vi "Configure Math.vi"(0 "VISA resource name":refnum<visa-resource-name>, 1 "Operation (0:None)":i32(ring) items=["None", "Min/Max", "Relative", "dB", "dBm", "Compare", "MX+B"], 2 "Relative Offset (0)":dbl, 3 "dBm Resistance (600 Ohms)":i32(ring)=600 items=["2"=2, "4"=4, "8"=8, "16"=16, "50"=50, "75"=75, "93"=93, "110"=110, "124"=124, "125"=125, "135"=135, "150"=150, "250"=250, "300"=300, "500"=500, "600"=600, "800"=800, "900"=900, "1000"=1000, "1200"=1200, "8000"=8000], 5 "dB Reference Point (0V)":dbl, 7 "Upper Limit (1)":dbl=1.0, 9 "Lower Limit (-1)":dbl=-1.0, 11 "error in (no error)":errorcluster, 12 "Scale Factor M (1)":dbl=1.0, 13 "Offset Factor B (0)":dbl) -> (4 "VISA resource name out":refnum<visa-resource-name>, 15 "error out":errorcluster)   [LabVIEW 2021, in "GWInstek  GDM8351.lvlib"]
doc: "Configures the math functions available on the instrument."
uses:
  <instrlib>/GWInstek  GDM8351/GWInstek  GDM8351.lvlib
panel:
  # "Relative Function"
  # "MX+B"
  # "DB Measurements"
  # "Compare(Limit)"
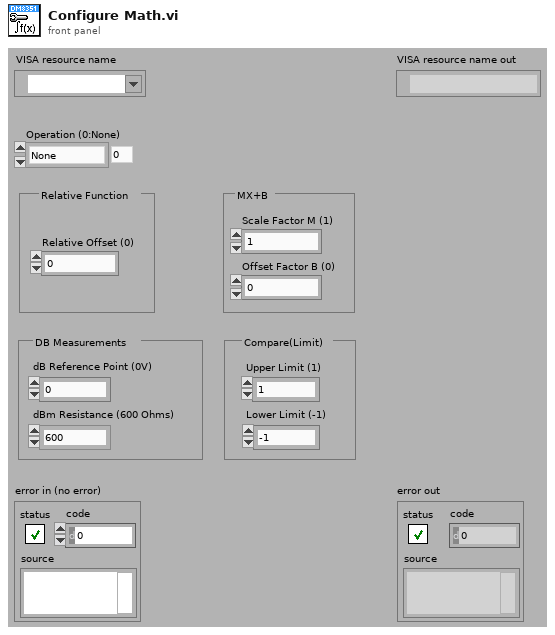
[diagram p1: front panel]
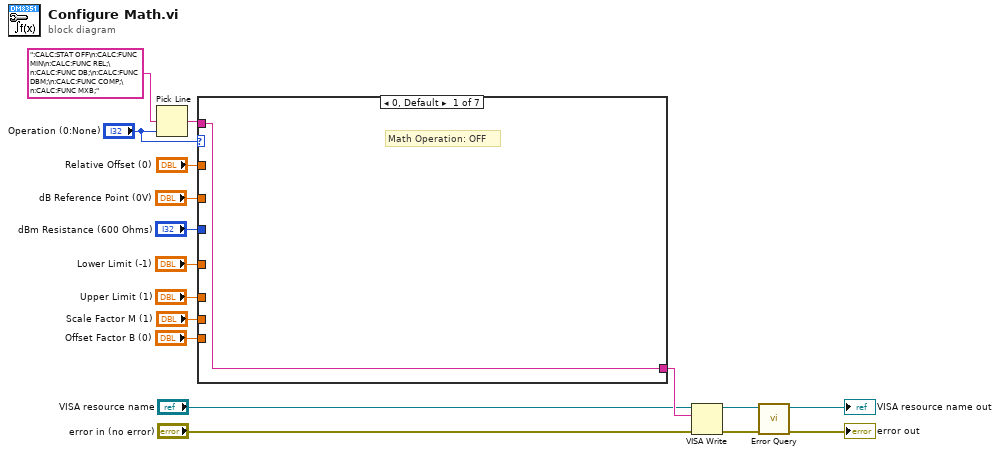
[diagram p0: block diagram]
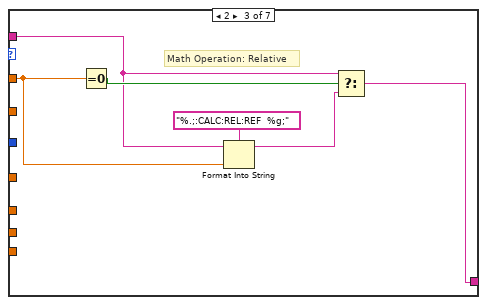
[diagram p3: hidden frame]
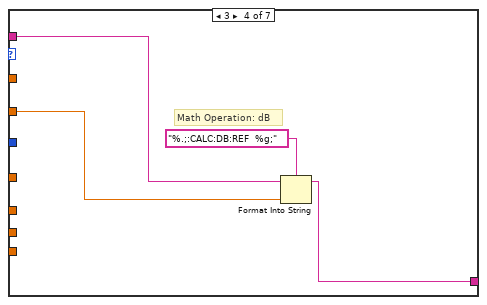
[diagram p4: hidden frame]
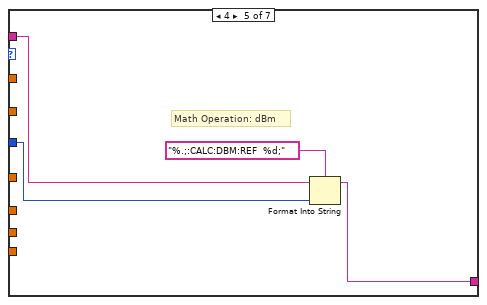
[diagram p5: hidden frame]
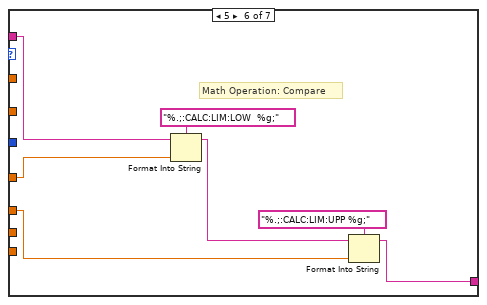
[diagram p6: hidden frame]
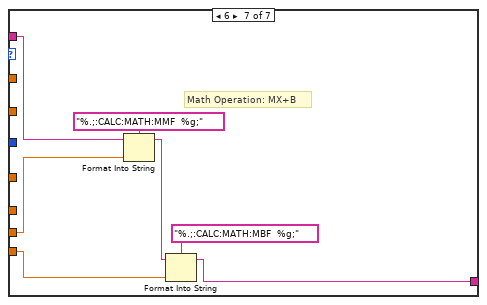
[diagram p7: hidden frame]
diagram:
  n1 = Pick Line(multi-line string=":CALC:STAT OFF\n:CALC:FUNC MIN\n:CALC:FUNC REL;\n:CALC:FUNC DB;\n:CALC:FUNC DBM;\n:CALC:FUNC COMP;\n:CALC:FUNC MXB;", line index="Operation (0:None)") -> (output string=w8:string)  [unwired: 1 in]
  n2 = case shown="0, Default" "Operation (0:None)" {
    tunnel: "Relative Offset (0)" -> [_ _ w22 _ _ _ _]
    tunnel: "dB Reference Point (0V)" -> [_ _ _ w29 _ _ _]
    tunnel: "dBm Resistance (600 Ohms)" -> [_ _ _ _ w31 _ _]
    tunnel: "Lower Limit (-1)" -> [_ _ _ _ _ w40 _]
    tunnel: "Upper Limit (1)" -> [_ _ _ _ _ w37 _]
    tunnel: "Scale Factor M (1)" -> [_ _ _ _ _ _ w47]
    tunnel: "Offset Factor B (0)" -> [_ _ _ _ _ _ w46]
    tunnel: w8 -> [w18 w19 w23 w28 w32 w39 w43]
    tunnel: [w18 w19 w20 w26 w30 w34 w41] -> w7
    frame 0, Default {
      # "Math Operation: OFF"
    }
    frame 1 {
      # "Math Operation: Min/Max"
    }
    frame 2 {
      # "Math Operation: Relative"
      n3 = Equal To 0?(x=w22) -> (x = 0?=w25:bool)
      n4 = Format Into String(format string="%.;:CALC:REL:REF  %g;", initial string=w23, w22) -> (resulting string=w21:string)  [unwired: 1 in, 1 out]
      n5 = Select(t=w23, s=w25, f=w21) -> (s? t:f=w20:string)
    }
    frame 3 {
      # "Math Operation: dB"
      n6 = Format Into String(format string="%.;:CALC:DB:REF  %g;", initial string=w28, w29) -> (resulting string=w26:string)  [unwired: 1 in, 1 out]
    }
    frame 4 {
      # "Math Operation: dBm"
      n7 = Format Into String(format string="%.;:CALC:DBM:REF  %d;", initial string=w32, w31) -> (resulting string=w30:string)  [unwired: 1 in, 1 out]
    }
    frame 5 {
      # "Math Operation: Compare"
      n8 = Format Into String(format string="%.;:CALC:LIM:LOW  %g;", initial string=w39, w40) -> (resulting string=w35:string)  [unwired: 1 in, 1 out]
      n9 = Format Into String(format string="%.;:CALC:LIM:UPP %g;", initial string=w35, w37) -> (resulting string=w34:string)  [unwired: 1 in, 1 out]
    }
    frame 6 {
      # "Math Operation: MX+B"
      n10 = Format Into String(format string="%.;:CALC:MATH:MMF  %g;", initial string=w43, w47) -> (resulting string=w42:string)  [unwired: 1 in, 1 out]
      n11 = Format Into String(format string="%.;:CALC:MATH:MBF  %g;", initial string=w42, w46) -> (resulting string=w41:string)  [unwired: 1 in, 1 out]
    }
  }
  n12 = VISA Write(VISA resource name="VISA resource name", write buffer=w7, error in (no error)="error in (no error)") -> (VISA resource name out=w4:refnum<visa-resource-name>, error out=w3:errorcluster)  [unwired: 1 out]
  n13 = call <instrlib>:"Error Query.vi"("error in (no error)"=w3, "VISA resource name"=w4) -> ("error out"=→"error out":errorcluster, "VISA resource name out"=→"VISA resource name out":refnum<visa-resource-name>)  [unwired: 6 in, 2 out]
